vi "checkTCPconnection.vi"(8 "error in (no error)":errorcluster, 11 "connection ID":refnum<k5>) -> (0 "error out":errorcluster, 3 "connection IDout":refnum<k5>)   [LabVIEW 2019, in "LifterTCP.lvclass"]
uses:
  LifterTCP.lvclass
panel:
  in  "address":string="192.168.24.142"
  in  "remote port or service name":u16=7776
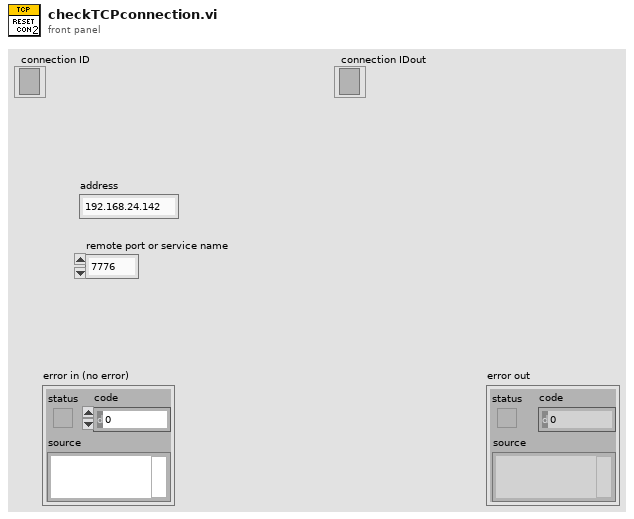
[diagram p1: front panel]
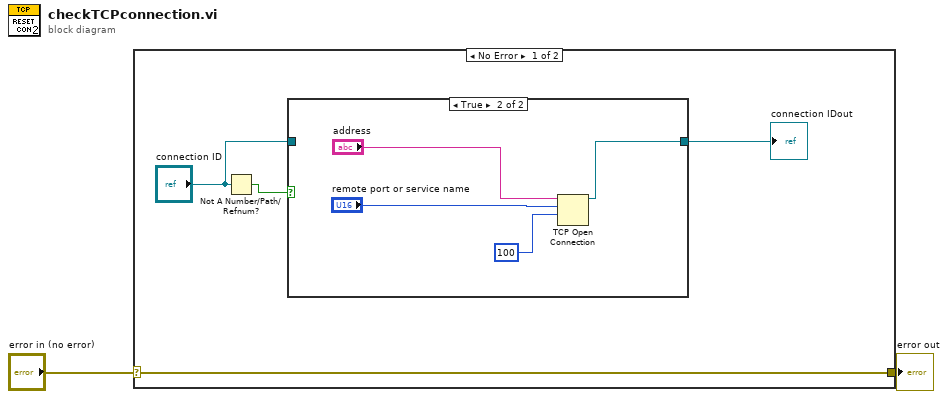
[diagram p0: block diagram]
diagram:
  n1 = case shown="No Error" "error in (no error)" {
    selector: "error in (no error)" -> [w6 w12]
    tunnel: [w6 w12] -> w1
    frame No Error {
      n2 = Not A Number/Path/Refnum?(number/path/refnum="connection ID") -> (NaN/Path/Refnum?=w5:bool)
      n3 = case shown="True" w5 {
        tunnel: [w7 w8] -> w4
        tunnel: "connection ID" -> [w7 _]
        frame False {
        }
        frame True {
          n4 = TCP Open Connection(address="address", remote port or service name="remote port or service name", timeout ms (60000)=100) -> (connection ID=w8:refnum<k5>)  [unwired: 2 in, 1 out]
        }
      }
      "connection IDout" <- w4
    }
    frame Error {
    }
  }
  "error out" <- w1
